vi "timetags2array.vi"(6 "show_flags":bool caption="Show Flags", 8 "start_read":u32[][](array[numeric]), 9 "stop_read":u32[][](array[numeric]), 10 "pixels/count":u32=5, 11 "timetags":u32[][](array[numeric])) -> (3 "photons_chart":u32[][](array[numeric]))   [LabVIEW 2018]
panel:
  out "q_stop":dbl[](array[numeric])
  out "q_start":dbl[](array[numeric])
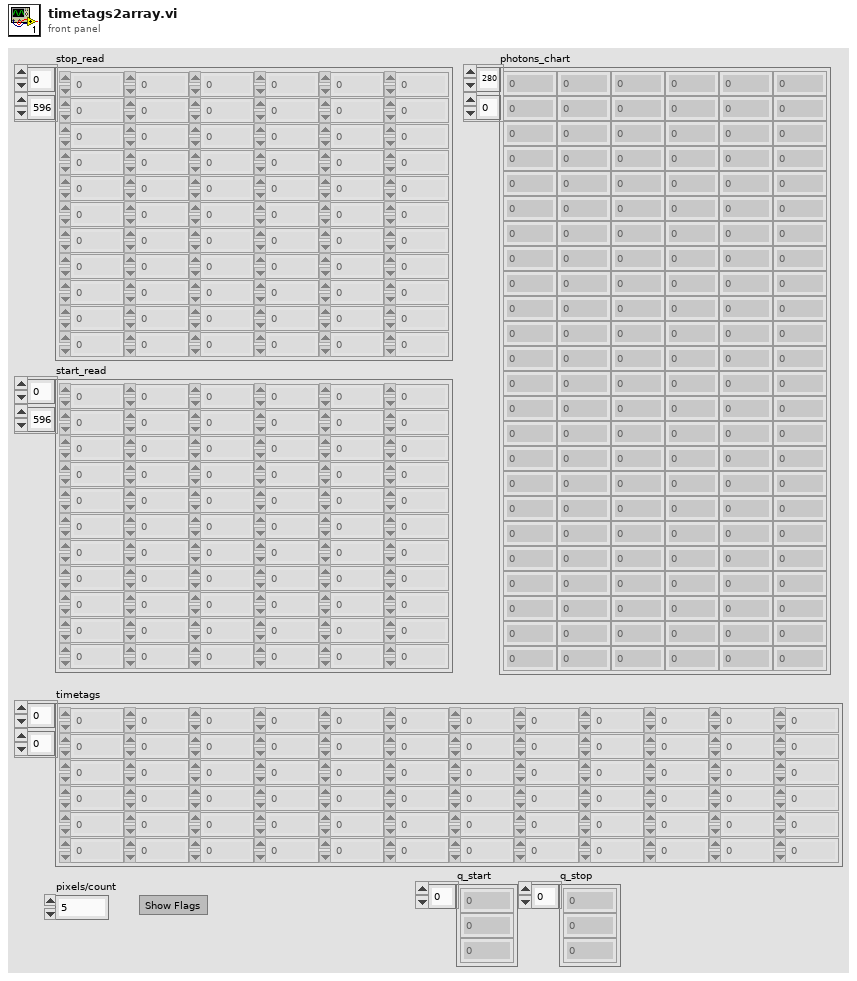
[diagram p1: front panel]
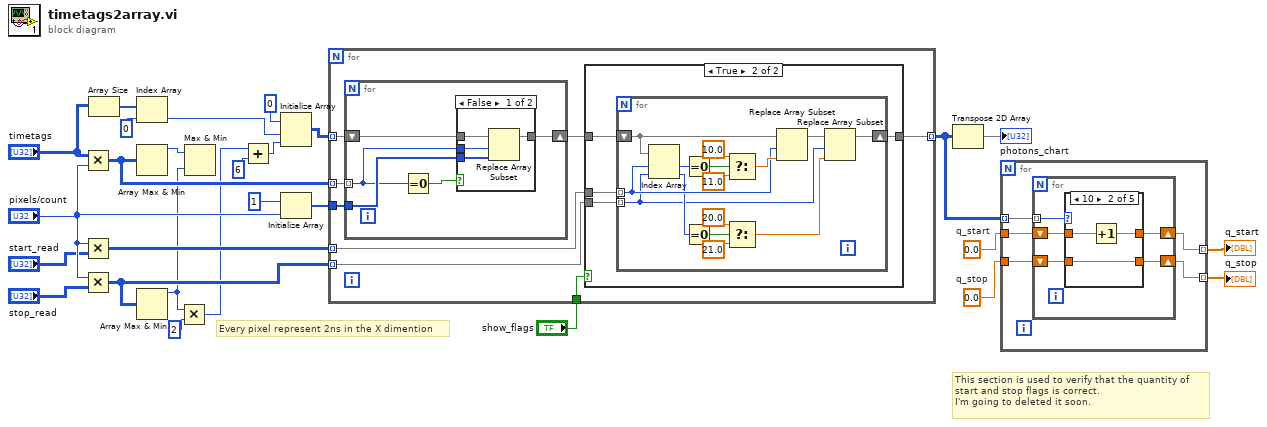
[diagram p0: block diagram]
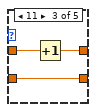
[diagram p3: hidden frame]
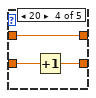
[diagram p4: hidden frame]
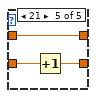
[diagram p5: hidden frame]
diagram:
  w10 = 0.0  # q_stop
  w11 = 0.0  # q_start
  # "This section is used to verify that the quantity of\nstart and stop flags is correct.\nI'm going to deleted it soon."
  # "Every pixel represent 2ns in the X dimention"
  n1 = Multiply(x="timetags", y="pixels/count") -> (x*y=w26:u32[][])
  n2 = Multiply(x="pixels/count", y="start_read") -> (x*y=w17:u32[][])
  n3 = Multiply(x="pixels/count", y="stop_read") -> (x*y=w7:u32[][])
  n4 = Array Size(array="timetags") -> (size(s)=w22:i32[])
  n5 = Index Array(array=w22, index=0) -> (element=w19:i32)
  n6 = Array Max & Min(array=w26) -> (max value=w6:u32)  [unwired: 3 out]
  n7 = Array Max & Min(array=w7) -> (max value=w1:u32)  [unwired: 3 out]
  n8 = Multiply(x=w1, y=u32 2) -> (x*y=w3:u32)
  n9 = Max & Min(x=w6, y=w1) -> ()  [unwired: 2 out]
  n10 = Add(x=w3, y=u32 6) -> (x+y=w20:u32)
  n11 = Initialize Array(u32 0 ("element"), w19, w20) -> (w18:u32[][])
  n12 = Initialize Array(u32 1 ("new element/subarray"), "pixels/count") -> (w24:u32[])
  n13 = for {
    tunnel: w18 -> [w35] mode=indexing
    tunnel: [w29] -> w8 mode=indexing
    tunnel: w26 -> [w33] mode=indexing
    tunnel: w17 -> [w32] mode=indexing
    tunnel: w7 -> [w31] mode=indexing
    tunnel: w24 -> [w30]
    tunnel: "show_flags" -> [w28]
    n14 = for {
      tunnel: w33 -> [w57] mode=indexing
      shift-right: [w59] -> w34
      shift-left: w35 -> [w60]
      tunnel: w30 -> [w58]
      n15 = Equal To 0?(x=w57) -> (x = 0?=w56:bool)
      n16 = case shown="False" w56 {
        tunnel: w60 -> [w64 w65]
        tunnel: [w63 w65] -> w59
        tunnel: w58 -> [w62 _]
        tunnel: w57 -> [w61 _]
        frame False {
          n17 = Replace Array Subset(array=w64, new element=w62, index=w61) -> (w63:u32[])
        }
        frame True {
        }
      }
    }
    n18 = case shown="True" w28 {
      tunnel: w34 -> [w36 w40]
      tunnel: w32 -> [_ w39]
      tunnel: w31 -> [_ w38]
      tunnel: [w36 w37] -> w29
      frame False {
      }
      frame True {
        n19 = for {
          shift-right: [w41] -> w37
          shift-left: w40 -> [w50]
          tunnel: w39 -> [w49] mode=indexing
          tunnel: w38 -> [w42] mode=indexing
          n20 = Index Array(array=w50, index #1=w49, index #2=w42) -> (element #1=w55:u32, element #2=w45:u32)
          n21 = Equal To 0?(x=w55) -> (x = 0?=w54:bool)
          n22 = Equal To 0?(x=w45) -> (x = 0?=w48:bool)
          n23 = Select(t=10.0, s=w54, f=11.0) -> (s? t:f=w51:dbl)
          n24 = Select(t=20.0, s=w48, f=21.0) -> (s? t:f=w43:dbl)
          n25 = Replace Array Subset(array=w50, new element=w51, index=w49) -> (w44:u32[])
          n26 = Replace Array Subset(array=w44, new element=w43, index=w42) -> (w41:u32[])
        }
      }
    }
  }
  n27 = Transpose 2D Array(2D array=w8) -> (transposed array=→"photons_chart":u32[][])
  n28 = for {
    tunnel: w8 -> [w70] mode=indexing
    tunnel: w11 -> [w69]
    tunnel: [w67] -> w9 mode=indexing
    tunnel: w10 -> [w68]
    tunnel: [w66] -> w5 mode=indexing
    n29 = for {
      tunnel: w70 -> [w71] mode=indexing
      shift-right: [w73] -> w67
      shift-left: w69 -> [w75]
      shift-right: [w72] -> w66
      shift-left: w68 -> [w74]
      n30 = case shown="10" w71 {
        tunnel: w75 -> [w77 w80 w83 w86 w87]
        tunnel: w74 -> [w76 w78 w81 w85 w89]
        tunnel: [w77 w79 w82 w86 w87] -> w73
        tunnel: [w76 w78 w81 w84 w88] -> w72
        frame 0, Default {
        }
        frame 10 {
          n31 = Increment(x=w80) -> (x+1=w79:dbl)
        }
        frame 11 {
          n32 = Increment(x=w83) -> (x+1=w82:dbl)
        }
        frame 20 {
          n33 = Increment(x=w85) -> (x+1=w84:dbl)
        }
        frame 21 {
          n34 = Increment(x=w89) -> (x+1=w88:dbl)
        }
      }
    }
  }
  "q_start" <- w9
  "q_stop" <- w5
